vi "Init.vi"(8 "error in (no error)":errorcluster, 10 "Eye Params":dbl[](array[numeric]), 11 "TrialBasedExperiment in":refnum<class "BehaviorClassification.lvclass">) -> (0 "error out":errorcluster, 3 "TrialBasedExperiment out":refnum<class "BehaviorClassification.lvclass">)   [LabVIEW 2010, in "BehaviorClassification.lvclass"]
uses:
  BehaviorClassification.lvclass
  MatlabExperiment/MatlabExperiment.lvclass
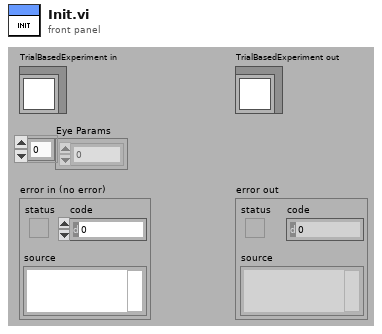
[diagram p1: front panel]
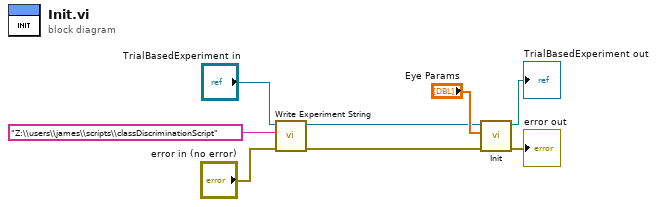
[diagram p0: block diagram]
diagram:
  n1 = call-dynamic "Write Experiment String.vi"("error in (no error)"="error in (no error)", "Experiment String"="Z:\\users\\james\\scripts\\classDiscriminationScript", "TrialBasedExperiment in"="TrialBasedExperiment in") -> ("error out"=w5:errorcluster, "TrialBasedExperiment out"=w1:refnum<class "BehaviorClassification.lvclass">)  [unwired: 7 in]
  n2 = call-parent "Init.vi"("error in (no error)"=w5, "Eye Params"="Eye Params", "TrialBasedExperiment in"=w1) -> ("error out"=→"error out":errorcluster, "TrialBasedExperiment out"=→"TrialBasedExperiment out":refnum<class "BehaviorClassification.lvclass">)  [unwired: 7 in]
